vi "Read Counter Double Wrapper.vi"(0 "Task map in":map{string, refnum<k21>}(c390), 5 "Message Data in":T2, 11 "error in (no error)":errorcluster) -> (4 "Task map out":map{string, refnum<k21>}(c390), 6 "Message Data Out":T1, 15 "error out":errorcluster)   [LabVIEW 2021, in "NI DAQmx_wrapper.lvlib"]
uses:
  NI DAQmx_wrapper.lvlib
  NI DAQmx_server/RPC Messages/nidaqmx_grpc_ReadCounterScalarF64Request.ctl
  NI DAQmx_server/RPC Messages/nidevice_grpc_Session_session/nidevice_grpc_Session_session.lvclass
  NI DAQmx_server/RPC Messages/nidevice_grpc_Session.ctl
  NI DAQmx_server/RPC Messages/nidaqmx_grpc_ReadCounterScalarF64Response.ctl
  NI DAQmx_server/RPC Messages/nidevice_grpc_Session_session/nidevice_grpc_Session_session.lvclass/nidevice_grpc_Session_session.ctl
  <vilib>/DAQmx/read.llb/DAQmx Read (Counter DBL 1Chan 1Samp).vi
  <vilib>/DAQmx/miscellaneous.llb/DAQmx Fill In Error Info.vi
  NI DAQmx_server/NI DAQmx_server.lvlib
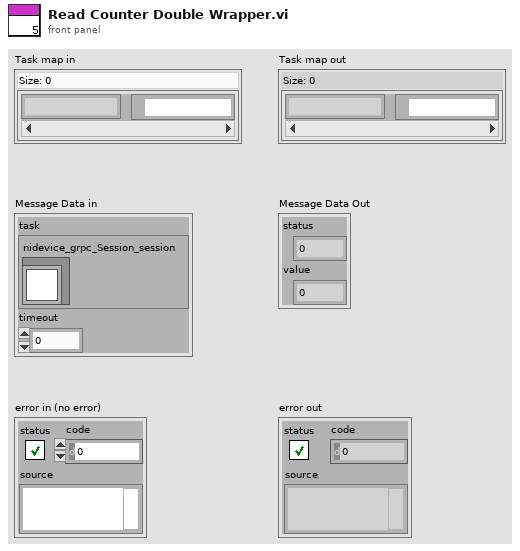
[diagram p1: front panel]
types:
  T1 = typedef "NI DAQmx_server.lvlib/nidaqmx_grpc_ReadCounterScalarF64Response.ctl" = cluster{"status":i32, "value":dbl}
  T2 = typedef "NI DAQmx_server.lvlib/nidaqmx_grpc_ReadCounterScalarF64Request.ctl" = cluster{"task":T3, "timeout":dbl}
  T3 = typedef "NI DAQmx_server.lvlib/nidevice_grpc_Session.ctl" = cluster{"nidevice_grpc_Session_session":refnum<class "nidevice_grpc_Session_session.lvclass">}
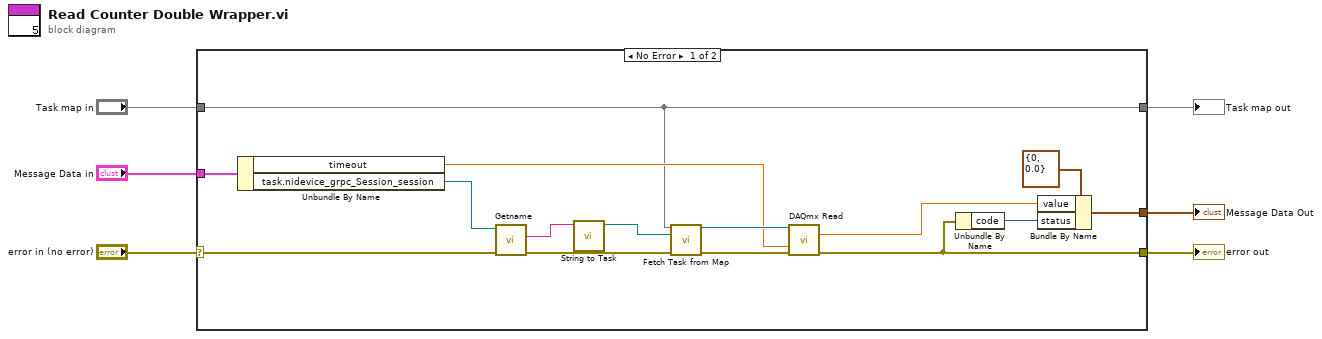
[diagram p0: block diagram]
diagram:
  n1 = case shown="No Error" "error in (no error)" {
    selector: "error in (no error)" -> [w17 w23]
    tunnel: [w9 w23] -> w5
    tunnel: "Task map in" -> [w7 w22]
    tunnel: [w7 w22] -> w3
    tunnel: "Message Data in" -> [w21 _]
    tunnel: [w8 _] -> w1
    frame No Error {
      n2 = Unbundle By Name(w21) -> ("timeout"=w13:dbl, "task.nidevice_grpc_Session_session"=w16:refnum<class "nidevice_grpc_Session_session.lvclass">)
      n3 = call "Getname.vi"("error in (no error)"=w17, "OneOfTemplate in"=w16) -> ("error out"=w18:errorcluster, "Get_Val"=w20:string)  [unwired: 7 in, 1 out]
      n4 = call "String to Task.vi"("Get_Val"=w20) -> ("Refnum out"=w19:refnum<k21>)  [unwired: 10 in]
      n5 = call "Fetch Task from Map.vi"("Task map in"=w7, "Task in"=w19, "error in (no error)"=w18) -> ("Task out"=w14:refnum<k21>, "error out"=w15:errorcluster)  [unwired: 11 in]
      n6 = call-poly <vilib>:"DAQmx Read.vi"("task/channels in"=w14, "timeout"=w13, "error in"=w15) -> ("data"=w10:dbl, "error out"=w9:errorcluster)  [unwired: 10 in, 1 out]
      n7 = Unbundle By Name(w9) -> ("code"=w12:i32)
      n8 = Bundle By Name(cluster=T1 {"status"=0, "value"=0.0} ("Message Data Out"), "value"=w10, "status"=w12) -> (w8:T1)
    }
    frame Error {
    }
  }
  "error out" <- w5
  "Task map out" <- w3
  "Message Data Out" <- w1
